vi "Test - Osciloscope - Inizializate 1.vi"(8 "error in (no error)":errorcluster, 11 "Module ID":i32) -> (0 "error out":errorcluster, 3 "Pass":bool)   [LabVIEW 2020]
doc: "_____\nCreated using DQMH Event Scripter 6.0.0.122."
uses:
  Libraries/Osciloscope/Osciloscope.lvlib
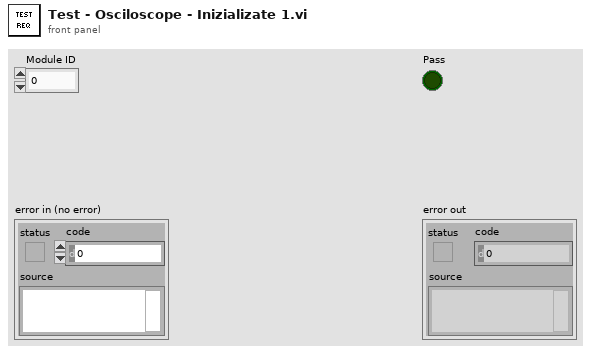
[diagram p1: front panel]
types:
  T1 = typedef "Osciloscope.lvlib/Broadcast Events--cluster.ctl" = cluster{"Module Did Init":refnum<user-event>, "Status Updated":refnum<user-event>, "Error Reported":refnum<user-event>, "Module Did Stop":refnum<user-event>, "Update Module Execution Status":refnum<user-event>, "Obtain Osciloscope Name":refnum<user-event>}
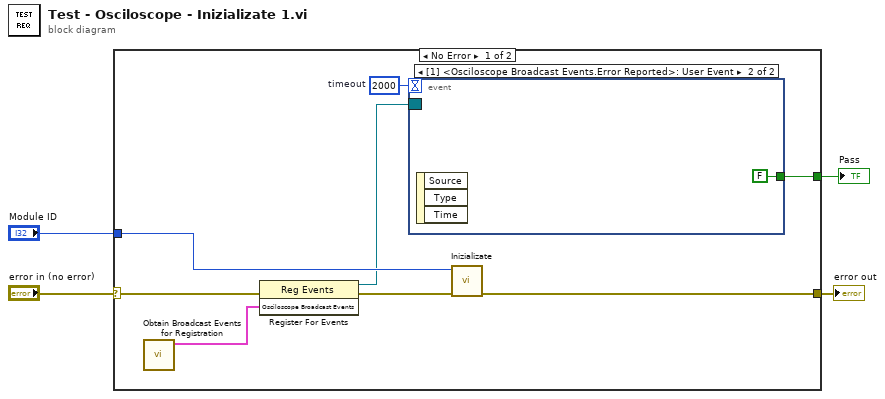
[diagram p0: block diagram]
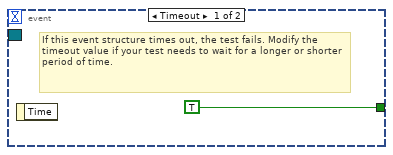
[diagram p2: hidden frame]
diagram:
  n1 = case shown="No Error" "error in (no error)" {
    selector: "error in (no error)" -> [w12 w15]
    tunnel: [w11 w15] -> w3
    tunnel: "Module ID" -> [w10 _]
    tunnel: [w5 _] -> w1
    frame No Error {
      w6 = 2000  # timeout
      n2 = call "Obtain Broadcast Events for Registration.vi"() -> ("Osciloscope Broadcast Events"=w8:T1)  [unwired: 9 in, 2 out]
      n3 = register-events(error in=w12, w8) -> (reference out=w7:refnum<event-registration>, error out=w9:errorcluster)  [unwired: 1 in]
      n4 = event shown="[1] <Osciloscope Broadcast Events.Error Reported>: User Event" {
        selector: w7 -> [_ _]
        dyn-events: _ -> [_ _]
        timeout: w6 -> [_ _]
        tunnel: [TRUE FALSE] -> w5
        event Timeout {
          # "If this event structure times out, the test fails. Modify the timeout value if your test needs to wait for a longer or shorter period of time."
          n5 = event-data() -> ()  [unwired: 1 in, 1 out]
        }
        event User Event {
          n6 = event-data() -> ()  [unwired: 1 in, 3 out]
        }
      }
      n7 = call "Inizializate.vi"("error in"=w9, "Module ID"=w10) -> ("error out"=w11:errorcluster)  [unwired: 9 in]
    }
    frame Error {
    }
  }
  "error out" <- w3
  "Pass" <- w1
